vi "Raycaster_SortObjects.vi"(11 "Decorations In":T1) -> (2 "Sorted Indexes":u8[](array[numeric]), 3 "Decorations Out":T1)   [LabVIEW 2020]
uses:
  Controls/Map_Objects.ctl
  Controls/Map_Object.ctl
  Controls/Map_Position.ctl
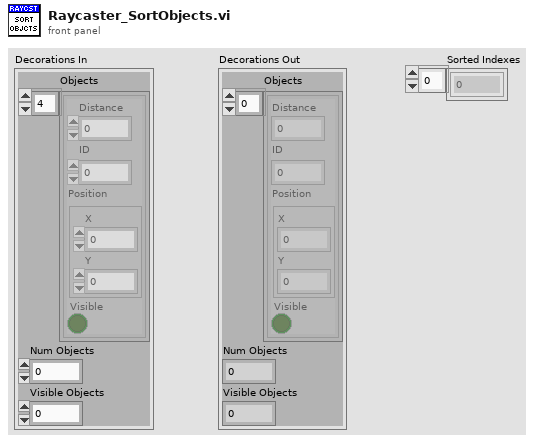
[diagram p1: front panel]
types:
  T1 = typedef "Map_Objects.ctl" = cluster{"Objects":T2[], "Num Objects":i16, "Visible Objects":i16}
  T2 = typedef "Map_Object.ctl" = cluster{"Distance":fxp<+/-,32,16>, "ID":u8, "Position":T3, "Visible":bool}
  T3 = typedef "Map_Position.ctl" = cluster{"X":fxp<+/-,32,16>, "Y":fxp<+/-,32,16>}
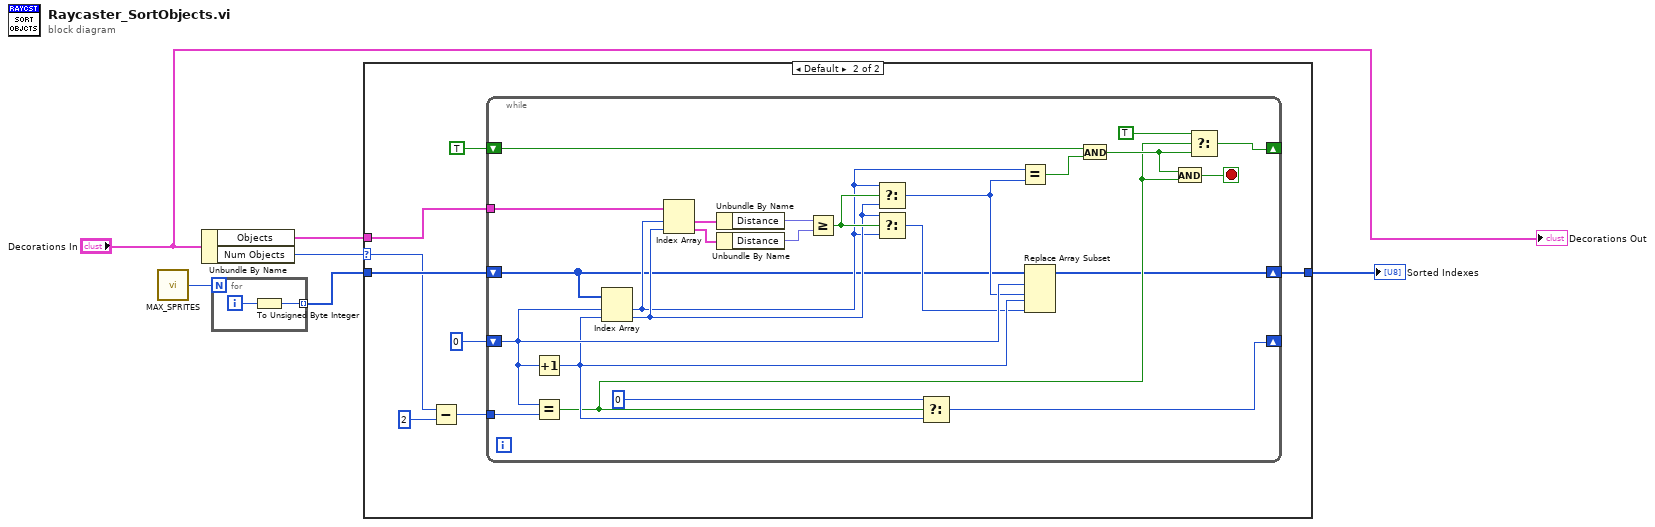
[diagram p0: block diagram]
diagram:
  n1 = call "MAX_SPRITES.vi"() -> ("MAX_SPRITES"=w2:u8)
  n2 = Unbundle By Name("Decorations In") -> ("Objects"=w3:T2[], "Num Objects"=w1:i16)
  n3 = for {
    N: w2 -> [_]
    tunnel: [w7] -> w5 mode=indexing
    i -> [w8]
    n4 = To Unsigned Byte Integer(number=w8) -> (unsigned 8bit integer=w7:u8)
  }
  n5 = case shown="Default" w1 {
    selector: w1 -> [_ w10]
    tunnel: w5 -> [w9 w17]
    tunnel: [w9 w16] -> w4
    tunnel: w3 -> [_ w15]
    frame ..1 {
    }
    frame Default {
      n6 = Subtract(x=w10, y=i16 2) -> (x-y=w14:i16)
      n7 = while {
        shift-right: [w18] -> w16
        shift-left: w17 -> [w19]
        shift-right: [w39] -> _
        shift-left: TRUE -> [w41]
        tunnel: w14 -> [w36]
        shift-right: [w34] -> _
        shift-left: i16 0 -> [w33]
        tunnel: w15 -> [w29]
        stop <- w37 stop-if-true
        n8 = Increment(x=w33) -> (x+1=w32:i16)
        n9 = Equal?(x=w33, y=w36) -> (x = y?=w31:bool)
        n10 = Index Array(array=w19, index #1=w33, index #2=w32) -> (element #1=w21:u8, element #2=w22:u8)
        n11 = Index Array(array=w29, index #1=w21, index #2=w22) -> (element #1=w28:T2, element #2=w27:T2)
        n12 = Unbundle By Name(w28) -> ("Distance"=w26:fxp<+/-,32,16>)
        n13 = Unbundle By Name(w27) -> ("Distance"=w25:fxp<+/-,32,16>)
        n14 = Greater Or Equal?(x=w26, y=w25) -> (x >= y?=w24:bool)
        n15 = Select(t=w21, s=w24, f=w22) -> (s? t:f=w23:u8)
        n16 = Select(t=w22, s=w24, f=w21) -> (s? t:f=w20:u8)
        n17 = Select(t=i16 0, s=w31, f=w32) -> (s? t:f=w34:i16)
        n18 = Equal?(x=w21, y=w23) -> (x = y?=w30:bool)
        n19 = Replace Array Subset(array=w19, new element #1=w23, index #1=w33, new element #2=w20, index #2=w32) -> (w18:u8[])
        n20 = And(x=w41, y=w30) -> (x .and. y?=w38:bool)
        n21 = And(x=w38, y=w31) -> (x .and. y?=w37:bool)
        n22 = Select(t=TRUE, s=w31, f=w38) -> (s? t:f=w39:bool)
      }
    }
  }
  "Sorted Indexes" <- w4
  "Decorations Out" <- "Decorations In"
